vi "Random Waveform Simulator.vi"(1 "Channel #":dbl, 2 "dt":dbl, 3 "# Points":i64) -> (0 "waveform out":waveform(dbl))   [LabVIEW 2021]
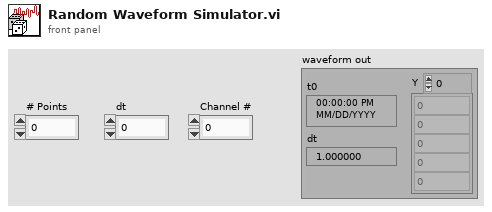
[diagram p1: front panel]
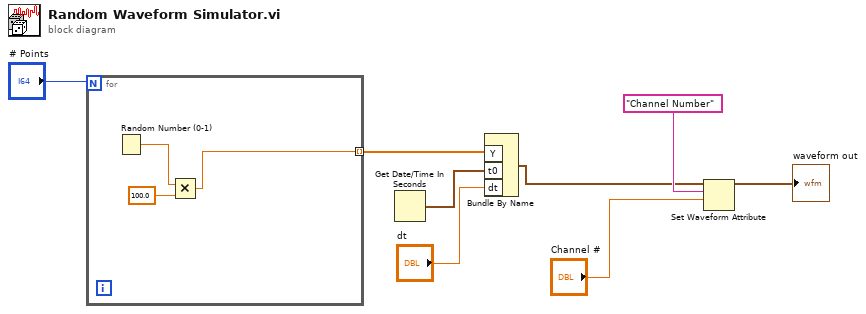
[diagram p0: block diagram]
diagram:
  n1 = for {
    N: "# Points" -> [_]
    tunnel: [w9] -> w5 mode=indexing
    n2 = Random Number (0-1)() -> (number: 0 to 1=w10:dbl)
    n3 = Multiply(x=w10, y=100.0) -> (x*y=w9:dbl)
  }
  n4 = Get Date/Time In Seconds() -> (seconds since 1Jan1904=w3:timestamp)
  n5 = Bundle By Name("Y"=w5, "t0"=w3, "dt"="dt") -> (w2:waveform(dbl))  [unwired: 1 in]
  n6 = Set Waveform Attribute(5:"Channel #", 6:"Channel Number", 7:w2) -> (3:→"waveform out":waveform(dbl))  [unwired: 1 in, 2 out]
